vi "Format Image.vi"(1 "Picture Color Type":T1, 4 "Picture Index":i32=-1, 5 "Measurement System":T2=enum."Metric", 6 "error in (no error)":errorcluster, 7 "Width":dbl=-1.0, 8 "Scale Factor":dbl=1.0, 9 "Height":dbl=-1.0, 10 "Report Ref In":T3) -> (0 "error out":errorcluster, 3 "Report Ref Out":T3)   [LabVIEW 2013, in "XCel Report Engine.lvlib"]
doc: "Changes the size or color presentation of an image in the active worksheet.\n\nPicture Index specifies the zero-based index of the image to format. A value of -1 selects the last image in the worksheet. Append Image.vi returns the index of each inserted image.\n\nScale Factor is applied to the current image dimensions. A value of 1 preserves the current size, 0.5 halves it, and 2 doubles it.\n\nHeight and Width optionally set explicit dimensions using the selected Measurement System. US values are interpreted in inches and Metric values in centimetres. A value of -1 leaves the corresponding dimension unchanged.\n\nColor Type controls the image color transformation. Automatic preserves the original colors and Grayscale applies a grayscale transformation. Other compatibility values are not supported by the current OpenXML backend.\n\nAn error is returned if the selected picture index does not exist or any formatting value is invalid."
uses:
  XCel Report Engine.lvlib
  C:/Users/m.santucci/Documents/ChatGPT/LV_REPORT_ENGINE/LV/DotNet/XCelReportEngine.dll
  LV/DotNet/XCelReportEngine.dll
  Controls/Report Ref.ctl
  Controls/Measurement System.ctl
  Controls/Picture Color Type.ctl
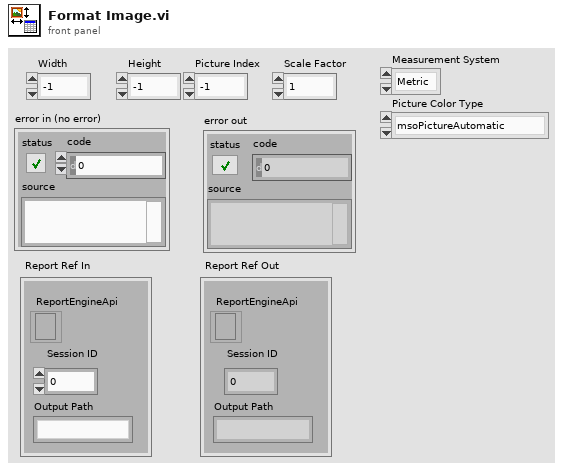
[diagram p1: front panel]
types:
  T1 = typedef "XCel Report Engine.lvlib/Picture Color Type.ctl" = enum32{"msoPictureAutomatic", "msoPictureMixed", "msoPictureGrayscale", "msoPictureBlack&White", "msoPictureWatermark"}
  T2 = typedef "XCel Report Engine.lvlib/Measurement System.ctl" = enum32{"US", "Metric"}
  T3 = typedef "XCel Report Engine.lvlib/Report Ref.ctl" = cluster{"Session ID":i32, "Output Path":string, "ReportEngineApi":refnum<k24>}
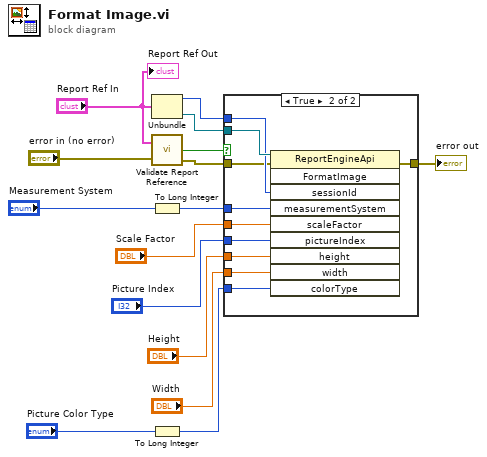
[diagram p0: block diagram]
diagram:
  n1 = Unbundle("Report Ref In") -> ("Session ID"=w13:i32, "ReportEngineApi"=w15:refnum<k24>)  [unwired: 1 out]
  n2 = call "Validate Report Reference.vi"("Report Ref In"="Report Ref In", "error in (no error)"="error in (no error)") -> ("Valid"=w1:bool, "error out"=w3:errorcluster)  [unwired: 1 out]
  n3 = To Long Integer(number="Measurement System") -> (32bit integer=w7:i32)
  n4 = To Long Integer(number="Picture Color Type") -> (32bit integer=w9:i32)
  n5 = case shown="True" w1 {
    tunnel: w15 -> [_ w26]
    tunnel: [w16 w25] -> w14
    tunnel: w13 -> [_ w24]
    tunnel: "Picture Index" -> [_ w23]
    tunnel: "Width" -> [_ w22]
    tunnel: w9 -> [_ w21]
    tunnel: w7 -> [_ w20]
    tunnel: "Height" -> [_ w19]
    tunnel: "Scale Factor" -> [_ w18]
    tunnel: w3 -> [w16 w17]
    frame False {
    }
    frame True {
      n6 = invoke class="ReportEngineApi" method="FormatImage"(reference=w26, error in=w17, "sessionId"=w24, "measurementSystem"=w20, "scaleFactor"=w18, "pictureIndex"=w23, "height"=w19, "width"=w22, "colorType"=w21) -> (error out=w25:errorcluster)  [unwired: 1 in, 9 out]
    }
  }
  "error out" <- w14
  "Report Ref Out" <- "Report Ref In"
